vi "wd_replaceInIndexCheck.vi"(6 "data type":T7, 8 "error in (no error)":errorcluster, 9 "value index":u64, 10 "channel index":u32, 11 "meta in":T1={"TargetFile"=path "", "StreamMode"=enum."File", "Append?"=FALSE, "ChunkSize"=0, "TimeColumnMode"=enum."Empty", "TimestampFormat"="", "AbsoluteTime?"=FALSE, "FileAttribute "={"Creator"="", "Title"="", "SheetName"=""}, "Column"=[], "FileRef"=refnum, "MemoryRef"=[], "RecordInfo"=[], " ChannelPreviousInfo"=[], "ChannelFirstRecord"=[], "PredefinedFormattedValueLength"=20, "DiskTemplate"={"XMLRef"=[refnum, refnum, refnum, refnum, refnum, refnum], "ZipPath"=path "", "MetaFile"={"Ref"=refnum, "NextRow"=0, "NextPosition"=0, "Block"=[]}, "TempFolder"=path ""}}) -> (0 "error out":errorcluster, 3 "meta out":T1={"TargetFile"=path "", "StreamMode"=enum."File", "Append?"=FALSE, "ChunkSize"=0, "TimeColumnMode"=enum."Empty", "TimestampFormat"="", "AbsoluteTime?"=FALSE, "FileAttribute "={"Creator"="", "Title"="", "SheetName"=""}, "Column"=[], "FileRef"=refnum, "MemoryRef"=[], "RecordInfo"=[], " ChannelPreviousInfo"=[], "ChannelFirstRecord"=[], "PredefinedFormattedValueLength"=20, "DiskTemplate"={"XMLRef"=[refnum, refnum, refnum, refnum, refnum, refnum], "ZipPath"=path "", "MetaFile"={"Ref"=refnum, "NextRow"=0, "NextPosition"=0, "Block"=[]}, "TempFolder"=path ""}})   [LabVIEW 2020, in "NI_ExcelFile.lvlib"]
uses:
  <vilib>/express/express shared/NI_ExcelFile/NI_ExcelFile.lvlib
  <vilib>/express/express shared/NI_ExcelFile/Ctrls/DataType.ctl
  <vilib>/express/express shared/NI_ExcelFile/Ctrls/MainData.ctl
  <vilib>/express/express shared/NI_ExcelFile/Ctrls/StreamMode.ctl
  <vilib>/express/express shared/NI_ExcelFile/Ctrls/TimeColumnMode.ctl
  <vilib>/express/express shared/NI_ExcelFile/Ctrls/FileAttribute.ctl
  <vilib>/express/express shared/NI_ExcelFile/Ctrls/Columns.ctl
  <vilib>/express/express shared/NI_ExcelFile/Ctrls/ColumnInfo.ctl
  <vilib>/express/express shared/NI_ExcelFile/Ctrls/wd_recordInfo.ctl
  <vilib>/express/express shared/NI_ExcelFile/Ctrls/disk_TemplateFile.ctl
  <vilib>/express/express shared/NI_ExcelFile/Ctrls/meta_file.ctl
  <vilib>/express/express shared/NI_ExcelFile/Ctrls/meta_Block.ctl
  <vilib>/express/express shared/NI_ExcelFile/Ctrls/meta_BlockType.ctl
  <vilib>/Utility/error.llb/Error Cluster From Error Code.vi
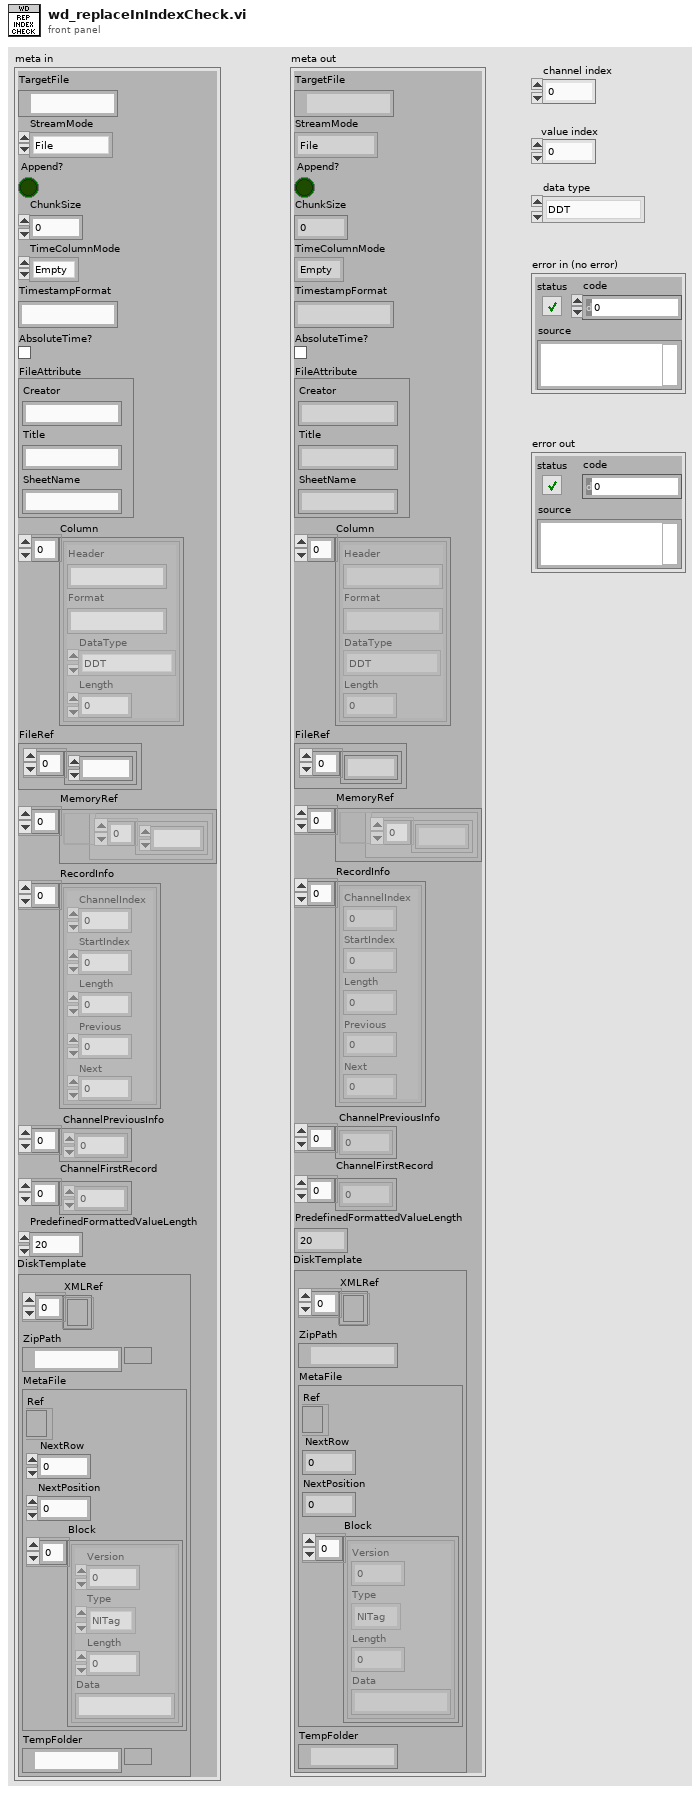
[diagram p1: front panel]
types:
  T1 = typedef "NI_ExcelFile.lvlib/MainData.ctl" = cluster{"TargetFile":path, "StreamMode":T2, "Append?":bool, "ChunkSize":u64, "TimeColumnMode":T3, "TimestampFormat":string, "AbsoluteTime?":bool, "FileAttribute ":T4, "Column":T5, "FileRef":refnum<k1>, "MemoryRef":refnum<data-value>[], "RecordInfo":T8[], " ChannelPreviousInfo":u32[], "ChannelFirstRecord":u32[], "PredefinedFormattedValueLength":i64, "DiskTemplate":T9}
  T2 = typedef "NI_ExcelFile.lvlib/StreamMode.ctl" = enum16{"File", "Memory"}
  T3 = typedef "NI_ExcelFile.lvlib/TimeColumnMode.ctl" = enum16{"Empty", "OnePerCh", "One"}
  T4 = typedef "NI_ExcelFile.lvlib/FileAttribute.ctl" = cluster{"Creator":string, "Title":string, "SheetName":string}
  T5 = typedef "NI_ExcelFile.lvlib/Columns.ctl" = T6[]
  T6 = typedef "NI_ExcelFile.lvlib/ColumnInfo.ctl" = cluster{"Header":string, "Format":string, "DataType":T7, "Length":u64}
  T7 = typedef "NI_ExcelFile.lvlib/DataType.ctl" = enum16{"DDT", "WFM", "Array of STR", "Array of DBL", "Array of I8", "Array of I16", "Array of I32", "Array of I64", "Array of SGL", "Array of U8", "Array of U16", "Array of U32", "Array of U64", "Array of Time"}
  T8 = typedef "NI_ExcelFile.lvlib/wd_recordInfo.ctl" = cluster{"ChannelIndex":u32, "StartIndex":u64, "Length":u64, "Previous":i32, "Next":i32}
  T9 = typedef "NI_ExcelFile.lvlib/disk_TemplateFile.ctl" = cluster{"XMLRef":refnum<file>[], "ZipPath":path, "MetaFile":T10, "TempFolder":path}
  T10 = typedef "NI_ExcelFile.lvlib/meta_file.ctl" = cluster{"Ref":refnum<file>, "NextRow":i32, "NextPosition":i64, "Block":T11[]}
  T11 = typedef "NI_ExcelFile.lvlib/meta_Block.ctl" = cluster{"Version":u16, "Type":T12, "Length":i32, "Data":string}
  T12 = typedef "NI_ExcelFile.lvlib/meta_BlockType.ctl" = enum16{"NITag", "File", "Column"}
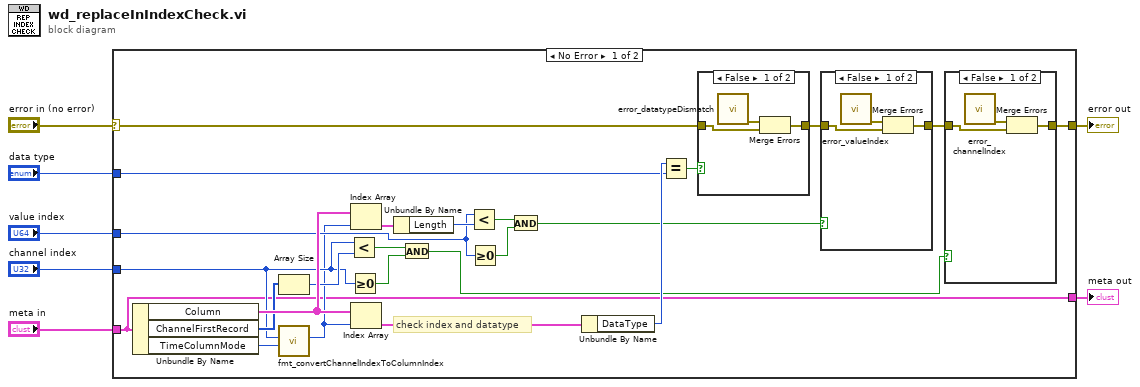
[diagram p0: block diagram]
diagram:
  n1 = case shown="No Error" "error in (no error)" {
    selector: "error in (no error)" -> [w10 w44]
    tunnel: "channel index" -> [w14 _]
    tunnel: "meta in" -> [w11 w45]
    tunnel: [w11 w45] -> w5
    tunnel: [w8 w44] -> w3
    tunnel: "value index" -> [w15 _]
    tunnel: "data type" -> [w16 _]
    frame No Error {
      # "check index and datatype"
      n2 = Unbundle By Name(w11) -> ("Column"=w27:T5, "ChannelFirstRecord"=w26:u32[], "TimeColumnMode"=w13:T3)
      n3 = Array Size(array=w26) -> (size(s)=w25:i32)
      n4 = call <vilib>:"fmt_convertChannelIndexToColumnIndex.vi"("TimeColumnMode"=w13, "channel index"=w14) -> ("data column index"=w12:i32)  [unwired: 8 in, 1 out]
      n5 = Less?(x=w14, y=w25) -> (x < y?=w21:bool)
      n6 = Greater Or Equal To 0?(x=w14) -> (x >= 0?=w20:bool)
      n7 = Index Array(array=w27, index=w12) -> (element=w28:T6)
      n8 = Index Array(array=w27, index=w12) -> (element=w30:T6)
      n9 = Unbundle By Name(w28) -> ("Length"=w29:u64)
      n10 = And(x=w21, y=w20) -> (x .and. y?=w19:bool)
      n11 = Less?(x=w15, y=w29) -> (x < y?=w24:bool)
      n12 = Greater Or Equal To 0?(x=w15) -> (x >= 0?=w23:bool)
      n13 = And(x=w24, y=w23) -> (x .and. y?=w22:bool)
      n14 = Unbundle By Name(w30) -> ("DataType"=w31:T7)
      n15 = Equal?(x=w31, y=w16) -> (x = y?=w17:bool)
      n16 = case shown="False" w17 {
        tunnel: w10 -> [w34 w35]
        tunnel: [w33 w35] -> w9
        frame False {
          n17 = call <vilib>:"error_datatypeDismatch.vi"() -> ("error out"=w32:errorcluster)  [unwired: 11 in]
          n18 = Merge Errors(w32, w34) -> (w33:errorcluster)
        }
        frame True {
        }
      }
      n19 = case shown="False" w22 {
        tunnel: w9 -> [w42 w43]
        tunnel: [w41 w43] -> w18
        frame False {
          n20 = call <vilib>:"error_valueIndex.vi"() -> ("error out"=w40:errorcluster)  [unwired: 11 in]
          n21 = Merge Errors(w40, w42) -> (w41:errorcluster)
        }
        frame True {
        }
      }
      n22 = case shown="False" w19 {
        tunnel: w18 -> [w38 w39]
        tunnel: [w37 w39] -> w8
        frame False {
          n23 = call <vilib>:"error_channelIndex.vi"() -> ("error out"=w36:errorcluster)  [unwired: 11 in]
          n24 = Merge Errors(w36, w38) -> (w37:errorcluster)
        }
        frame True {
        }
      }
    }
    frame Error {
    }
  }
  "meta out" <- w5
  "error out" <- w3
